vi "Actor Core.vi"(8 "error in":errorcluster, 11 "Nested in":refnum<class "Logger Level.lvclass">) -> (0 "error out":errorcluster, 3 "Actor out":refnum<class "Actor.lvclass">)   [LabVIEW 2020, in "Logger Level.lvlib" / "Logger Level.lvclass"]
doc: "(<B>Filename</B>: Actor Framework.lvlib:Actor.lvclass:Actor Core.vi)\n\nReceives messages to the actor, reacts to them, and initiates any error handling that may shut the actor down.\n\nDescendant classes may override this VI to append parallel tasks for the actor to complete while it handles messages. Overrides use the Call Parent Method node."
uses:
  Logger Level.lvclass
  <vilib>/ActorFramework/Actor/Actor.lvclass
  <vilib>/ActorFramework/Stop Msg/Stop Msg.lvclass
  Logger/Logger/Logger.lvclass
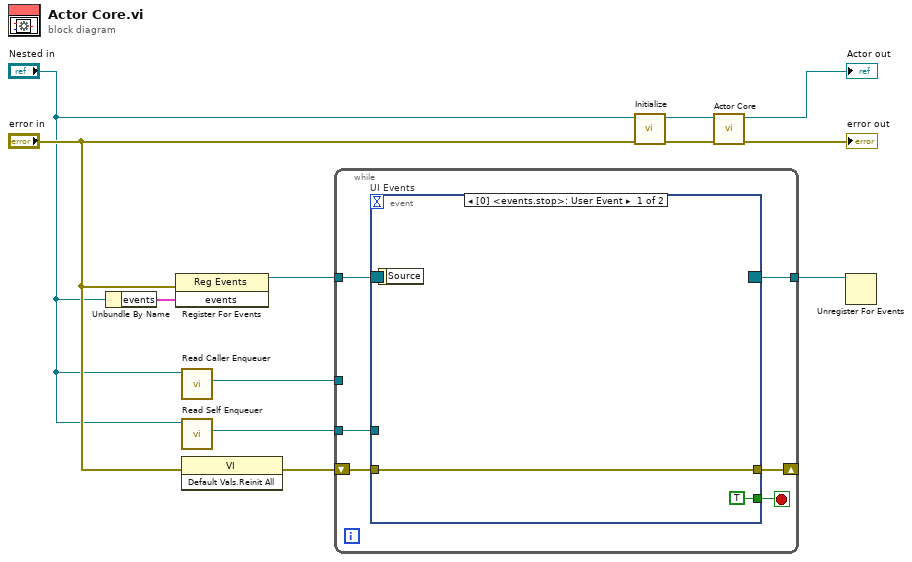
[diagram p0: block diagram]
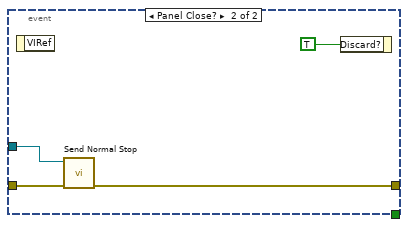
[diagram p2: hidden frame]
diagram:
  n1 = Unbundle By Name("Nested in") -> ("events"=w9:cluster{"stop":refnum<user-event>})
  n2 = register-events ("Main Register for Events")(error in="error in", w9) -> (reference out=w10:refnum<event-registration>)  [unwired: 1 in, 1 out]
  n3 = call <vilib>:"Read Caller Enqueuer.vi"("Actor"="Nested in") -> ("Caller Enqueuer"=w6:refnum<class "Message Enqueuer.lvclass">)  [unwired: 10 in]
  n4 = call <vilib>:"Read Self Enqueuer.vi"("Actor"="Nested in") -> ("Self Enqueuer"=w7:refnum<class "Message Enqueuer.lvclass">)  [unwired: 10 in]
  n5 = invoke class="VI" method="Default Vals.Reinit All"(error in="error in") -> (error out=w5:errorcluster)  [unwired: 2 in, 2 out]
  n6 = while {
    tunnel: w10 -> [w18]
    tunnel: [w16] -> w8
    tunnel: w7 -> [w15]
    tunnel: w6 -> [_]
    shift-right: [w13] -> _
    shift-left: w5 -> [w14]
    stop <- w17 stop-if-true
    n7 = event "UI Events" shown="[0] <events.stop>: User Event" {
      selector: w18 -> [_ _]
      dyn-events: [_ _] -> w16
      timeout: _ -> [_ _]
      tunnel: [TRUE _] -> w17
      tunnel: w15 -> [_ w23]
      tunnel: w14 -> [w20 w22]
      tunnel: [w20 w21] -> w13
      event User Event {
        n8 = event-data() -> ()  [unwired: 1 in, 1 out]
      }
      event Panel Close? {
        n9 = event-data() -> ()  [unwired: 1 in, 1 out]
        n10 = call <vilib>:"Send Normal Stop.vi"("error in (no error)"=w22, "Message Enqueuer"=w23) -> ("error out"=w21:errorcluster)  [unwired: 9 in]
        n11 = event-data("Discard?"=TRUE) -> ()  [unwired: 1 in, 1 out]
      }
    }
  }
  n12 = call "Initialize.vi"("error in (no error)"="error in", "View Template in"="Nested in") -> ("error out"=w4:errorcluster, "View Template out"=w3:refnum<class "Logger Level.lvclass">)  [unwired: 8 in]
  n13 = call-parent "Actor Core.vi"("error in"=w4, "Logger in"=w3) -> ("error out"=→"error out":errorcluster, "Actor out"=→"Actor out":refnum<class "Actor.lvclass">)  [unwired: 8 in]
  n14 = Unregister For Events(event registration refnum=w8) -> ()  [unwired: 1 in, 1 out]
